vi "QueueRequestForFile.vi"(0 "SettingsFileList in":refnum<class "SettingsFileList.lvclass">, 1 "Path":path, 2 "ProjectName":string, 3 "FileName":string, 4 "MD5 (optional)":string, 5 "error in (no error)":errorcluster) -> (14 "SettingsFileList out":refnum<class "SettingsFileList.lvclass">, 19 "error out":errorcluster)   [LabVIEW 2018, in "feGEM DataPacker.lvlib" / "SettingsFileList.lvclass"]
uses:
  SettingsFileList.lvclass
  SettingsFileList.lvclass/SettingsFileList.ctl
  SettingsFile.lvclass/SettingsFile.ctl
  SettingsFile.lvclass
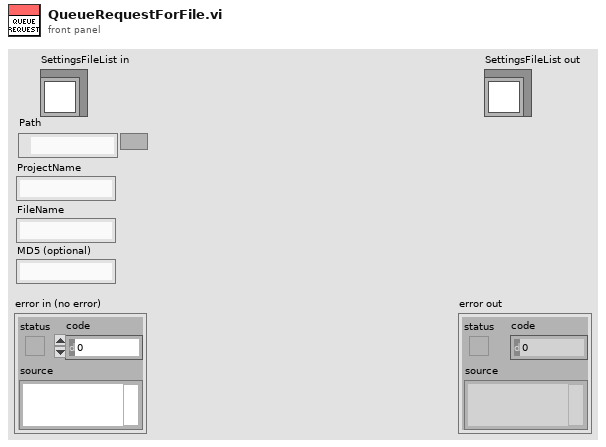
[diagram p1: front panel]
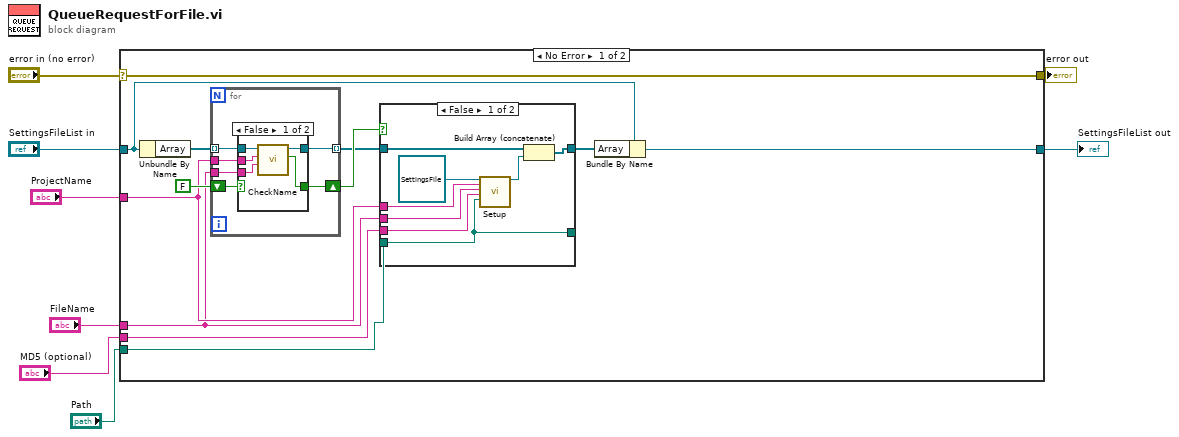
[diagram p0: block diagram]
diagram:
  n1 = case shown="No Error" "error in (no error)" {
    selector: "error in (no error)" -> [w20 w44]
    tunnel: [w20 w44] -> w7
    tunnel: [w17 w45] -> w5
    tunnel: "SettingsFileList in" -> [w18 w45]
    tunnel: "Path" -> [w14 _]
    tunnel: "ProjectName" -> [w10 _]
    tunnel: "FileName" -> [w9 _]
    tunnel: "MD5 (optional)" -> [w15 _]
    frame No Error {
      n2 = Unbundle By Name(w18) -> ("Array"=w19:refnum<class "SettingsFile.lvclass">[])
      n3 = for {
        tunnel: w19 -> [w36] mode=indexing
        tunnel: [w35] -> w12 mode=indexing
        shift-right: [w32] -> w13
        shift-left: FALSE -> [w31]
        tunnel: w10 -> [w34]
        tunnel: w9 -> [w33]
        n4 = case shown="False" w31 {
          selector: w31 -> [_ w42]
          tunnel: w36 -> [w41 w43]
          tunnel: [w40 w43] -> w35
          tunnel: w34 -> [w39 _]
          tunnel: w33 -> [w38 _]
          tunnel: [w37 w42] -> w32
          frame False {
            n5 = call "CheckName.vi"("FileName"=w38, "ProjectName"=w39, "SettingsFile in"=w41) -> ("Boolean"=w37:bool, "SettingsFile out"=w40:refnum<class "SettingsFile.lvclass">)  [unwired: 6 in, 1 out]
          }
          frame True {
          }
        }
      }
      n6 = case shown="False" w13 {
        tunnel: w10 -> [w27 _]
        tunnel: w9 -> [w26 _]
        tunnel: w15 -> [w25 _]
        tunnel: w14 -> [w21 w29]
        tunnel: w12 -> [w24 w30]
        tunnel: [w22 w30] -> w11
        tunnel: [w21 w29] -> _
        frame False {
          n7 = call "Setup.vi"("SettingsFile in"=refnum<class "SettingsFile.lvclass"> refnum ("SettingsFile.lvclass"), "ProjectName"=w27, "FileName"=w26, "MD5 (optional)"=w25, "Path"=w21) -> ("SettingsFile out"=w23:refnum<class "SettingsFile.lvclass">)  [unwired: 13 in, 1 out]
          n8 = Build Array (concatenate)(w24, w23) -> (w22:refnum<class "SettingsFile.lvclass">[])
        }
        frame True {
        }
      }
      n9 = Bundle By Name(cluster=w18, "Array"=w11) -> (w17:refnum<class "SettingsFileList.lvclass">)
    }
    frame Error {
    }
  }
  "error out" <- w7
  "SettingsFileList out" <- w5
